vi "sub_numpy-arange.vi"(9 "step":dbl, 10 "max":dbl, 11 "start":dbl) -> (3 "x+y":dbl[](array[numeric]))   [LabVIEW 2019]
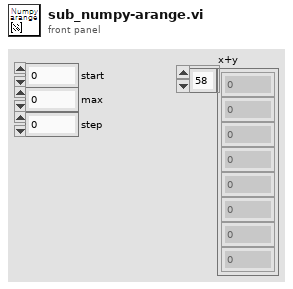
[diagram p1: front panel]
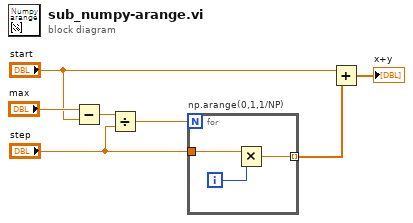
[diagram p0: block diagram]
diagram:
  n1 = Subtract(x="max", y="start") -> (x-y=w4:dbl)
  n2 = Divide(x=w4, y="step") -> (x/y=w2:dbl)
  n3 = for "np.arange(0,1,1/NP)" {
    N: w2 -> [_]
    tunnel: "step" -> [w9]
    tunnel: [w8] -> w7 mode=indexing
    i -> [w10]
    n4 = Multiply(x=w9, y=w10) -> (x*y=w8:dbl)
  }
  n5 = Add(x="start", y=w7) -> (x+y=→"x+y":dbl[])
